vi "QueryData.vi"(8 "TimeoutLengthSeconds":sgl, 9 "NumBytesExpected":u32, 10 "Message":u8[](array[numeric]), 11 "Handle":u32) -> (0 "Timeout":bool, 1 "Return Array":u8[](array[numeric]), 2 "Bytes Read":u32, 3 "FT_Status":u32(ring) items=["FT_OK", "FT_INVALID_HANDLE", "FT_DEVICE_NOT_FOUND", "FT_DEVICE_NOT_OPENED", "FT_IO_ERROR", "FT_INSUFFICIENT_RESOURCES", "FT_INVALID_PARAMETER", "FT_INVALID_BAUD_RATE", "FT_DEVICE_NOT_OPENED_FOR_ERASE", "FT_DEVICE_NOT_OPENED_FOR_WRITE", "FT_FAILED_TO_WRITE_DEVICE", "FT_EEPROM_READ_FAILED", "FT_EEPROM_WRITE_FAILED", "FT_EEPROM_ERASE_FAILED", "FT_EEPROM_NOT_PRESENT", "FT_EEPROM_NOT_PROGRAMMED", "FT_INVALID_ARGS", "FT_NOT_SUPPORTED", "FT_OTHER_ERROR"])   [LabVIEW 2013]
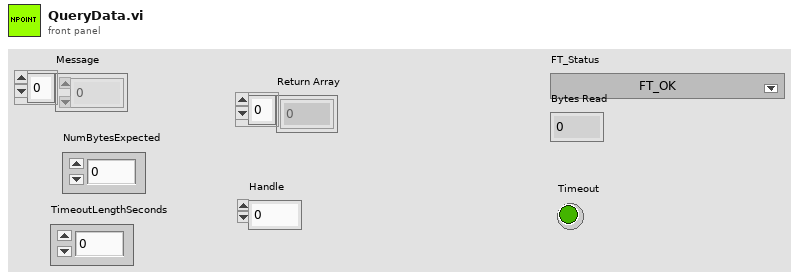
[diagram p1: front panel]
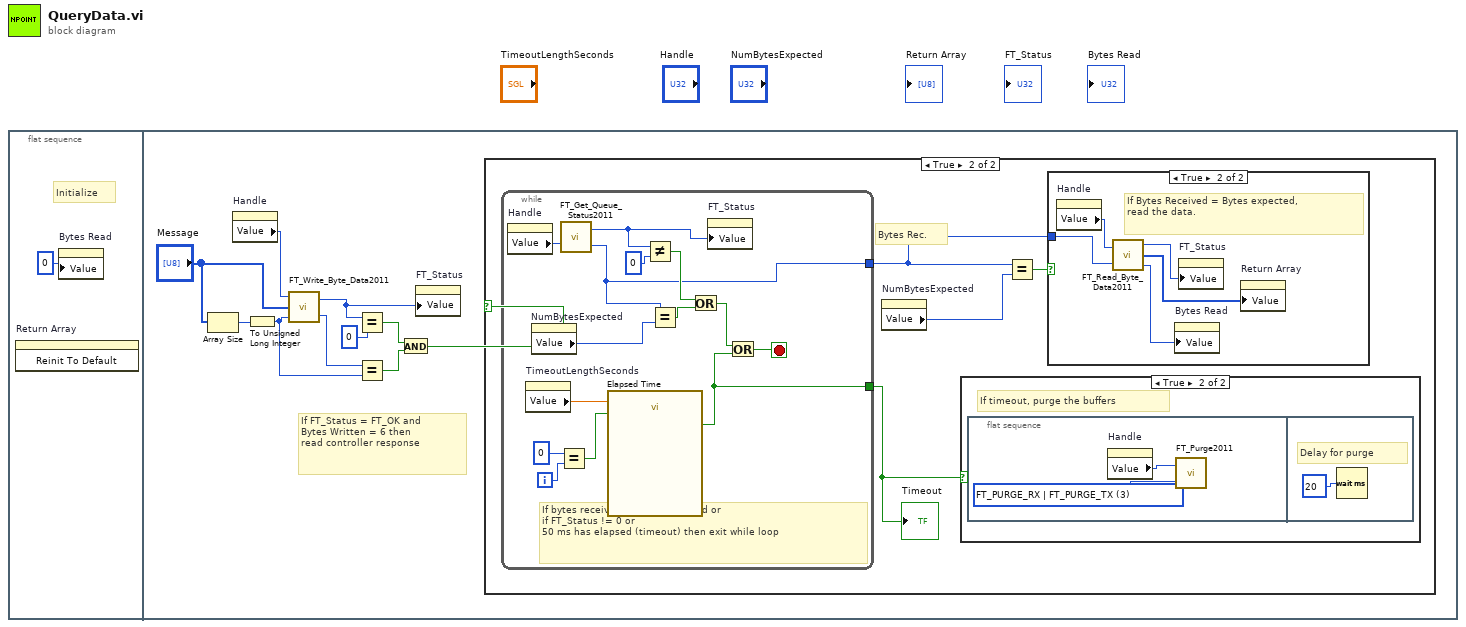
[diagram p0: block diagram]
diagram:
  n1 = flat-sequence {
    frame #0 {
      # "Initialize"
      n2 = invoke on="Return Array" class="Arr (strict)" method="Reinit To Default"() -> ()  [unwired: 3 in, 3 out]
      n3 = property on="Bytes Read" class="DigNum (strict)"("Value"=u32 0 ("Bytes Read")) -> ()  [unwired: 2 in, 2 out]
    }
    frame #1 {
      # "If FT_Status = FT_OK and\nBytes Written = 6 then\nread controller response"
      n4 = Array Size(array="Message") -> (size(s)=w11:i32)
      n5 = property on="Handle" class="DigNum (strict)"() -> ("Value"=w2:u32)  [unwired: 2 in, 2 out]
      n6 = To Unsigned Long Integer(number=w11) -> (unsigned 32bit integer=w4:u32)
      n7 = call "FT_Write_Byte_Data2011.vi"("Bytes To Write"=w4, "Buffer"="Message", "Handle"=w2) -> ("Bytes Written"=w6:u32, "FT_Status"=w3:u32)
      n8 = Equal?(x=w3, y=u32 0) -> (x = y?=w9:bool)
      n9 = Equal?(x=w6, y=w4) -> (x = y?=w10:bool)
      n10 = And(x=w9, y=w10) -> (x .and. y?=w8:bool)
      n11 = property on="FT_Status" class="Ring (strict)"("Value"=w3) -> ()  [unwired: 2 in, 2 out]
      n12 = case shown="True" w8 {
        frame False {
        }
        frame True {
          # "Bytes Rec."
          n13 = while {
            tunnel: [w29] -> w14
            tunnel: [w28] -> w12
            i -> [w37]
            stop <- w30 stop-if-true
            # "If bytes received = bytes expected or\nif FT_Status != 0 or\n50 ms has elapsed (timeout) then exit while loop"
            n14 = property on="Handle" class="DigNum (strict)"() -> ("Value"=w25:u32)  [unwired: 2 in, 2 out]
            n15 = property on="TimeoutLengthSeconds" class="DigNum (strict)"() -> ("Value"=w24:sgl)  [unwired: 2 in, 2 out]
            n16 = property on="NumBytesExpected" class="DigNum (strict)"() -> ("Value"=w27:u32)  [unwired: 2 in, 2 out]
            n17 = Equal?(x=0, y=w37) -> (x = y?=w35:bool)
            n18 = call "FT_Get_Queue_Status2011.vi"("Handle"=w25) -> ("FT_Status"=w26:u32, "Bytes Waiting"=w29:u32)
            n19 = call "Elapsed Time"("Time Target (s)"=w24, "Reset"=w35) -> ("Time has Elapsed"=w28:bool)  [unwired: 10 in, 7 out]
            n20 = Not Equal?(x=w26, y=u32 0) -> (x != y?=w33:bool)
            n21 = Equal?(x=w29, y=w27) -> (x = y?=w32:bool)
            n22 = Or(x=w33, y=w32) -> (x .or. y?=w31:bool)
            n23 = property on="FT_Status" class="Ring (strict)"("Value"=w26) -> ()  [unwired: 2 in, 2 out]
            n24 = Or(x=w31, y=w28) -> (x .or. y?=w30:bool)
          }
          "Timeout" <- w12
          n25 = property on="NumBytesExpected" class="DigNum (strict)"() -> ("Value"=w13:u32)  [unwired: 2 in, 2 out]
          n26 = case shown="True" w12 {
            frame False {
            }
            frame True {
              # "If timeout, purge the buffers"
              n27 = flat-sequence {
                frame #0 {
                  w16 = u32 3 items=["FT_PURGE_RX"=1, "FT_PURGE_TX"=2, "FT_PURGE_RX | FT_PURGE_TX"=3] ("Purge Flags")
                  n28 = property on="Handle" class="DigNum (strict)"() -> ("Value"=w17:u32)  [unwired: 2 in, 2 out]
                  n29 = call "FT_Purge2011.vi"("Purge Flags"=w16, "Handle"=w17) -> ()  [unwired: 1 out]
                }
                frame #1 {
                  # "Delay for purge"
                  n30 = Wait (ms)(milliseconds to wait=u32 20) -> ()  [unwired: 1 out]
                }
              }
            }
          }
          n31 = Equal?(x=w14, y=w13) -> (x = y?=w15:bool)
          n32 = case shown="True" w15 {
            tunnel: w14 -> [_ w23]
            frame False {
            }
            frame True {
              # "If Bytes Received = Bytes expected,\nread the data."
              n33 = property on="Handle" class="DigNum (strict)"() -> ("Value"=w19:u32)  [unwired: 2 in, 2 out]
              n34 = call "FT_Read_Byte_Data2011.vi"("Handle"=w19, "Bytes To Read"=w23) -> ("FT_Status"=w21:u32, "Read Data"=w22:u8[], "Bytes Read"=w20:u32)
              n35 = property on="Bytes Read" class="DigNum (strict)"("Value"=w20) -> ()  [unwired: 2 in, 2 out]
              n36 = property on="FT_Status" class="Ring (strict)"("Value"=w21) -> ()  [unwired: 2 in, 2 out]
              n37 = property on="Return Array" class="Arr (strict)"("Value"=w22) -> ()  [unwired: 2 in, 2 out]
            }
          }
        }
      }
    }
  }
